vi "FGV_ITC.vi"(5 "error in (no error)":errorcluster, 7 "ItemIndex":T1, 13 "Action":T2) -> (6 "error out":errorcluster, 8 "ItemsToChange":T1[](array[typedef]))   [LabVIEW 2009]
doc: "Function Globle Variable stores the index numbers."
uses:
  Controls/directions.ctl
  Controls/ItemIndex.ctl
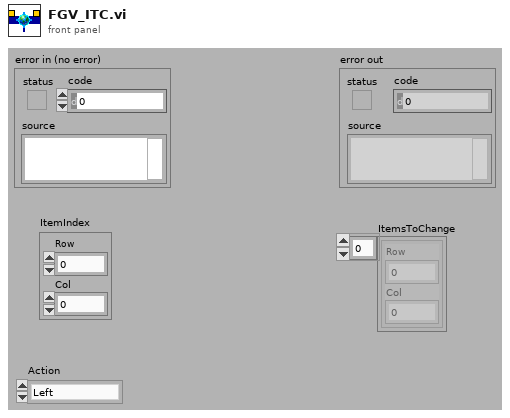
[diagram p1: front panel]
types:
  T1 = typedef "ItemIndex.ctl" = cluster{"Row":i32, "Col":i32}
  T2 = typedef "directions.ctl" = enum16{"Left", "Right", "Top", "Bottom", "TopLeft", "TopRight", "BottomLeft", "BottomRight", "ClearAll", "ReadAll"}
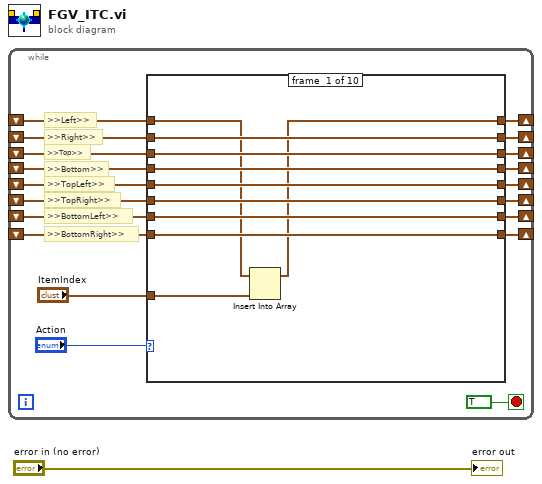
[diagram p0: block diagram]
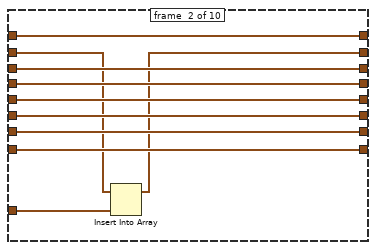
[diagram p2: hidden frame]
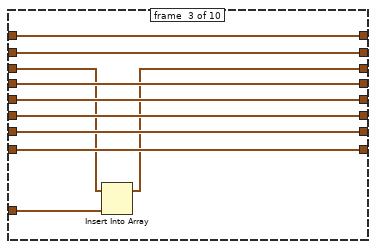
[diagram p3: hidden frame]
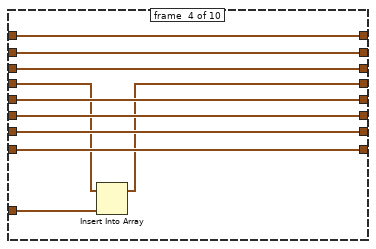
[diagram p4: hidden frame]
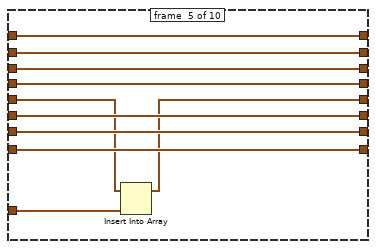
[diagram p5: hidden frame]
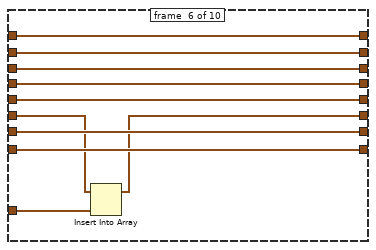
[diagram p6: hidden frame]
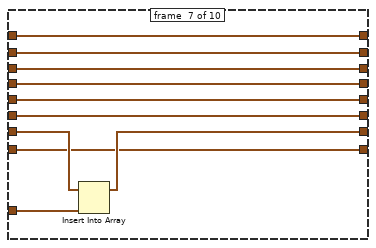
[diagram p7: hidden frame]
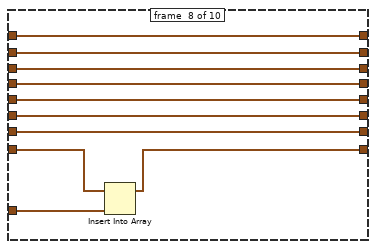
[diagram p8: hidden frame]
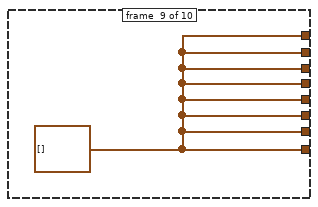
[diagram p9: hidden frame]
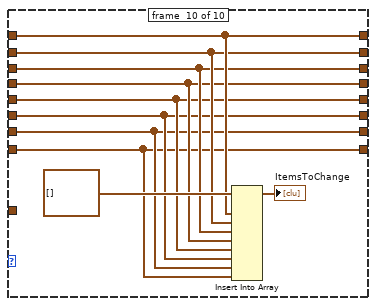
[diagram p10: hidden frame]
diagram:
  n1 = while {
    shift-right: [w11] -> _
    shift-left: _ -> [w19]
    shift-right: [w10] -> _
    shift-left: _ -> [w18]
    shift-right: [w9] -> _
    shift-left: _ -> [w17]
    shift-right: [w8] -> _
    shift-left: _ -> [w16]
    shift-right: [w7] -> _
    shift-left: _ -> [w15]
    shift-right: [w6] -> _
    shift-left: _ -> [w14]
    shift-right: [w5] -> _
    shift-left: _ -> [w13]
    shift-right: [w4] -> _
    shift-left: _ -> [w12]
    stop <- TRUE stop-if-true
    # ">>BottomRight>>"
    # ">>BottomLeft>>"
    # ">>TopRight>>"
    # ">>TopLeft>>"
    # ">>Bottom>>"
    # ">>Top>>"
    # ">>Right>>"
    # ">>Left>>"
    n2 = case shown="\"ReadAll\"" "Action" {
      tunnel: w19 -> [w23 w33 w50 w60 w70 w80 w90 w100 _ w110]
      tunnel: w18 -> [w30 w32 w49 w59 w69 w79 w89 w99 _ w109]
      tunnel: w17 -> [w29 w40 w42 w58 w68 w78 w88 w98 _ w108]
      tunnel: w16 -> [w28 w39 w48 w52 w67 w77 w87 w97 _ w107]
      tunnel: w15 -> [w27 w38 w47 w57 w62 w76 w86 w96 _ w106]
      tunnel: w14 -> [w26 w37 w46 w56 w66 w72 w85 w95 _ w105]
      tunnel: w13 -> [w25 w36 w45 w55 w65 w75 w83 w94 _ w104]
      tunnel: w12 -> [w24 w35 w44 w54 w64 w74 w81 w92 _ w103]
      tunnel: [w21 w33 w50 w60 w70 w80 w90 w100 w101 w110] -> w11
      tunnel: [w30 w31 w49 w59 w69 w79 w89 w99 w101 w109] -> w10
      tunnel: [w29 w40 w41 w58 w68 w78 w88 w98 w101 w108] -> w9
      tunnel: [w28 w39 w48 w51 w67 w77 w87 w97 w101 w107] -> w8
      tunnel: [w27 w38 w47 w57 w61 w76 w86 w96 w101 w106] -> w7
      tunnel: [w26 w37 w46 w56 w66 w71 w85 w95 w101 w105] -> w6
      tunnel: [w25 w36 w45 w55 w65 w75 w82 w94 w101 w104] -> w5
      tunnel: [w24 w35 w44 w54 w64 w74 w81 w91 w101 w103] -> w4
      tunnel: "ItemIndex" -> [w22 w34 w43 w53 w63 w73 w84 w93 _ _]
      frame #0 {
        n3 = Insert Into Array(array=w23, new element=w22) -> (w21:T1[])  [unwired: 1 in]
      }
      frame #1 {
        n4 = Insert Into Array(array=w32, new element=w34) -> (w31:T1[])  [unwired: 1 in]
      }
      frame #2 {
        n5 = Insert Into Array(array=w42, new element=w43) -> (w41:T1[])  [unwired: 1 in]
      }
      frame #3 {
        n6 = Insert Into Array(array=w52, new element=w53) -> (w51:T1[])  [unwired: 1 in]
      }
      frame #4 {
        n7 = Insert Into Array(array=w62, new element=w63) -> (w61:T1[])  [unwired: 1 in]
      }
      frame #5 {
        n8 = Insert Into Array(array=w72, new element=w73) -> (w71:T1[])  [unwired: 1 in]
      }
      frame #6 {
        n9 = Insert Into Array(array=w83, new element=w84) -> (w82:T1[])  [unwired: 1 in]
      }
      frame #7 {
        n10 = Insert Into Array(array=w92, new element=w93) -> (w91:T1[])  [unwired: 1 in]
      }
      frame #8 {
        w101 = T1[] [] ("appended array")
      }
      frame #9 {
        n11 = Insert Into Array(array=T1[] [] ("appended array"), new element #1=w110, new element #2=w109, new element #3=w108, new element #4=w107, new element #5=w106, new element #6=w105, new element #7=w104, new element #8=w103) -> (→"ItemsToChange":T1[])  [unwired: 1 in]
      }
    }
  }
  "error out" <- "error in (no error)"
